vi "Aktualizacja wyglądu mapy.vi"(7 "Położenie robota":T1, 9 "Skalowanie i kolory":T2={"Polozenie 1"={"X"=265, "Y"=265}, "  Wybór \nznacznika"=FALSE, "   Polozenie 2"={"X"=358, "Y"=265}, "   Blokada \nznaczników"=FALSE, "Kolor  znaczników"=16774930, "Grubość \nznaczników"=2, "Wyznaczanie odległości"=enum."Odległość pomiędzy znacznikami", "Współrzędne geograficzne 1"="", "Współrzędne geograficzne 2"="", "Odl. pomiędzy znacznikami [m]"=15.0}, 10 "Właściwości mapy":T4={"Przesunięcie mapy"={"X"=0, "Y"=0}, "Długość piksela w metrach"=0.19634281539316645, "Zoom mapy"=1.0, "Wpisane punkty na\nliście współrzędnych"=12271, "Zaznaczony punkt"=15663118, "Układ współrzędnych"=0, "Kierunek ruchu robota"=15663118, "Początkowe położenie robota"=15663118, "Trasa robota"=0, "Ostatni zaznaczony punkt na mapie"={"X"=0, "Y"=0}, "Draw Area Size"={"Width"=0, "Height"=0}} {"Zoom mapy" scale=0.2..4.0}, 11 "Mapa":picture) -> (3 "Przesunięta mapa":picture)   [LabVIEW 2012, in "Biblioteka moduł map v3.lvlib" / "Obsługa grafiki mapy.lvlib"]
doc: "Dorysowanie punktu startowego, osi położenia robota, zaznaczonego punktu oraz punktów z listy współrzędnych."
uses:
  <vilib>/Utility/miscctls.llb/LVBoundsTypeDef.ctl
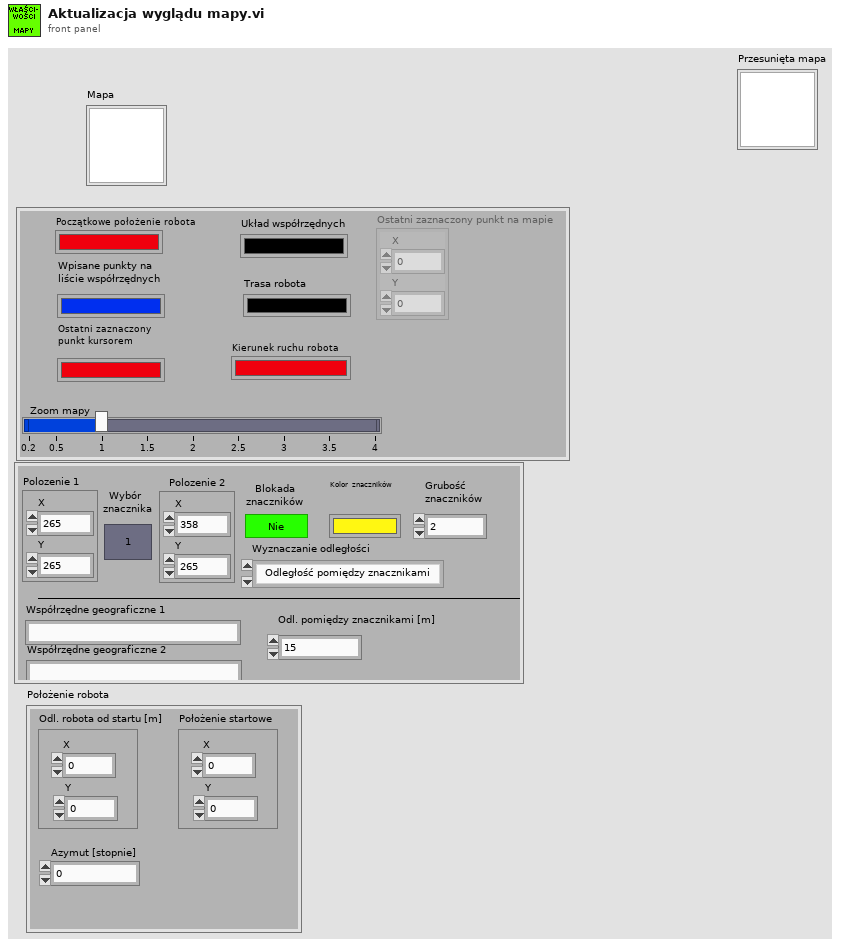
[diagram p1: front panel]
types:
  T1 = cluster{"Odl. robota od startu [m]":cluster{"X":dbl, "Y":dbl}, "Położenie startowe":cluster{"X":i32, "Y":i32}, "Azymut [stopnie]":dbl}
  T2 = cluster{"Polozenie 1":cluster{"X":i32, "Y":i32}, "  Wybór \nznacznika":bool, "   Polozenie 2":cluster{"X":i32, "Y":i32}, "   Blokada \nznaczników":bool, "Kolor  znaczników":u32, "Grubość \nznaczników":u32, "Wyznaczanie odległości":enum16{"Współrzędne geograficzne", "Odległość pomiędzy znacznikami"}, "Współrzędne geograficzne 1":string, "Współrzędne geograficzne 2":string, "Odl. pomiędzy znacznikami [m]":dbl}
  T3 = typedef "LVBoundsTypeDef.ctl" = cluster{"Width":u32, "Height":u32}
  T4 = cluster{"Przesunięcie mapy":cluster{"X":i16, "Y":i16}, "Długość piksela w metrach":dbl, "Zoom mapy":sgl, "Wpisane punkty na\nliście współrzędnych":u32, "Zaznaczony punkt":u32, "Układ współrzędnych":u32, "Kierunek ruchu robota":u32, "Początkowe położenie robota":u32, "Trasa robota":u32, "Ostatni zaznaczony punkt na mapie":cluster{"X":i32, "Y":i32}, "Draw Area Size":T3}
  T5 = cluster{"Szerokość (px)":i16, "Wysokość (px)":i16}
  T6 = cluster{"Położenie":cluster{"Pixel x":i16, "Pixel y":i16}, "Kolor punktu":u32, "Rozmiar punktu":u32, "Nazwa punktu":string}
  T7 = cluster{"Kolor skali":u32, "Odległość siatki od startu [px]":cluster{"X [m]":i32, "Y [m]":i32}, "Poł. startowe":cluster{"Piksel x":i32, "Piksel y":i32}}
  T8 = cluster{"Położenie  środka":cluster{"Pixel x":i16, "Pixel y":i16}, "Kolor ":u32, "Grubość  ":u32}
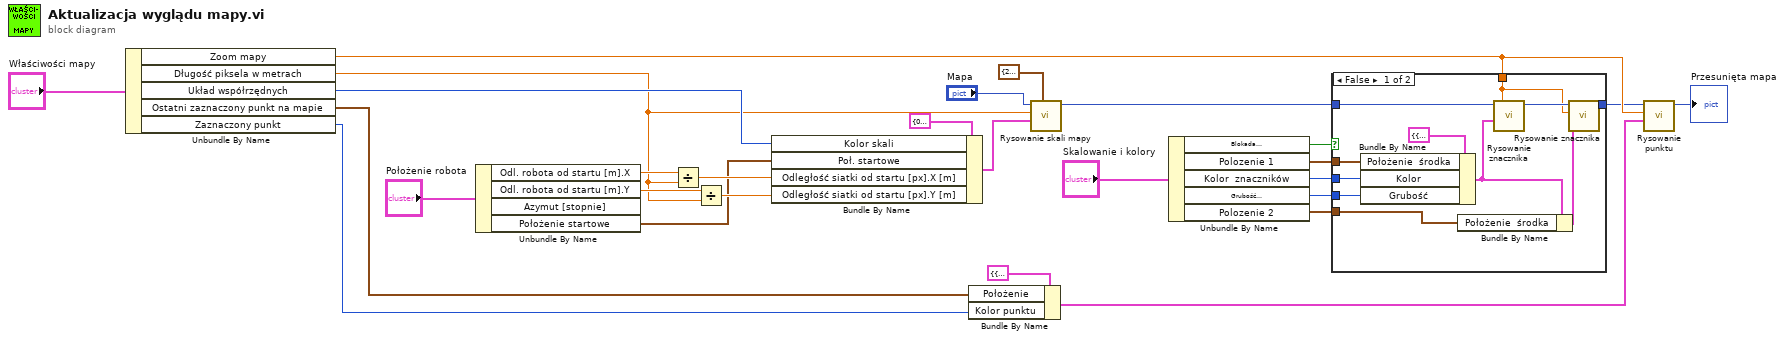
[diagram p0: block diagram]
diagram:
  n1 = Unbundle By Name("Właściwości mapy") -> ("Zoom mapy"=w13:sgl, "Długość piksela w metrach"=w12:dbl, "Układ współrzędnych"=w25:u32, "Ostatni zaznaczony punkt na mapie"=w2:cluster{"X":i32, "Y":i32}, "Zaznaczony punkt"=w1:u32)
  n2 = Unbundle By Name("Położenie robota") -> ("Odl. robota od startu [m].X"=w21:dbl, "Odl. robota od startu [m].Y"=w20:dbl, "Położenie startowe"=w3:cluster{"X":i32, "Y":i32})  [unwired: 1 out]
  n3 = Divide(x=w21, y=w12) -> (x/y=w11:dbl)
  n4 = Divide(x=w20, y=w12) -> (x/y=w10:dbl)
  n5 = Bundle By Name(cluster=T7 {"Kolor skali"=0, "Odległość siatki od startu [px]"={"X [m]"=61, "Y [m]"=-20}, "Poł. startowe"={"Piksel x"=246, "Piksel y"=243}} ("Parametry"), "Kolor skali"=w25, "Poł. startowe"=w3, "Odległość siatki od startu [px].X [m]"=w11, "Odległość siatki od startu [px].Y [m]"=w10) -> (w23:T7)
  n6 = Bundle By Name(cluster=T6 {"Położenie"={"Pixel x"=0, "Pixel y"=0}, "Kolor punktu"=0, "Rozmiar punktu"=2, "Nazwa punktu"=""} ("Punkt na mapie"), "Położenie"=w2, "Kolor punktu"=w1) -> (w14:T6)
  n7 = call "Rysowanie skali mapy.vi"("Rozmiar obszaru widocznej mapy"=T5 {"Szerokość (px)"=200, "Wysokość (px)"=200}, "Parametry"=w23, "Długość piksela w metrach"=w12, "Obraz wejściowy"="Mapa") -> ("Obraz wyjściowy"=w8:picture)  [unwired: 7 in]
  n8 = Unbundle By Name("Skalowanie i kolory") -> ("Blokada \nznaczników"=w9:bool, "Polozenie 1"=w19:cluster{"X":i32, "Y":i32}, "Kolor  znaczników"=w18:u32, "Grubość \nznaczników"=w17:u32, "Polozenie 2"=w16:cluster{"X":i32, "Y":i32})
  n9 = case shown="False" w9 {
    tunnel: [w38 w39] -> w4
    tunnel: w19 -> [w30 _]
    tunnel: w18 -> [w37 _]
    tunnel: w17 -> [w36 _]
    tunnel: w16 -> [w29 _]
    tunnel: w8 -> [w35 w39]
    tunnel: w13 -> [w28 _]
    frame False {
      n10 = Bundle By Name(cluster=T8 {"Położenie  środka"={"Pixel x"=358, "Pixel y"=265}, "Kolor "=16774930, "Grubość  "=2} ("Znacznik na mapie"), "Położenie  środka"=w30, "Kolor"=w37, "Grubość"=w36) -> (w32:T8)
      n11 = Bundle By Name(cluster=w32, "Położenie  środka"=w29) -> (w31:T8)
      n12 = call "Rysowanie znacznika.vi"("Znacznik na mapie"=w32, "Zoom mapy"=w28, "Mapa terenu"=w35) -> ("Mapa z wprowadzonym znacznikiem"=w34:picture)  [unwired: 8 in]
      n13 = call "Rysowanie znacznika.vi"("Znacznik na mapie"=w31, "Zoom mapy"=w28, "Mapa terenu"=w34) -> ("Mapa z wprowadzonym znacznikiem"=w38:picture)  [unwired: 8 in]
    }
    frame True {
    }
  }
  n14 = call "Rysowanie punktu.vi"("Punkt na mapie"=w14, "Zoom mapy"=w13, "Mapa terenu"=w4) -> ("Mapa z wprowadzonym punktem"=→"Przesunięta mapa":picture)  [unwired: 8 in]
